vi "DualMotorControlExample.vi"() -> ()   [LabVIEW 2019, in "CubeMarsBLDClib.lvlib"]
uses:
  CubeMarsBLDClib.lvlib
  MotorParameters.ctl
  Reference.ctl
  MotorType.ctl
  ReadMotorData.ctl
  <vilib>/myRIO/Common/Instrument Driver Framework/myRIO v1.0/UART/vis/myRIO v1.0 Close UART.vi
  <vilib>/myRIO/Common/Instrument Driver Framework/Utilities/vis/FPGA Ref Manager.vi
  <vilib>/myRIO/Common/Instrument Driver Framework/myRIO v1.0/myRIO v1.0 Reset FPGA.vi
  <vilib>/myRIO/Common/Instrument Driver Framework/myRIO v1.0/IRQ/vis/myRIO v1.0 IRQ Info FGV.vi
  <vilib>/myRIO/Common/Instrument Driver Framework/myRIO v1.0/IRQ/vis/myRIO v1.0 Timer IRQ Info FGV.vi
  <vilib>/myRIO/Common/Instrument Driver Framework/myRIO v1.0/IRQ/vis/myRIO v1.0 ISR Agent.vi
  <vilib>/myRIO/Instrument Drivers/Utilities/vis/Reset Index.vi
  <vilib>/myRIO/Common/Instrument Driver Framework/myRIO v1.0/Resource Manager/vis/myRIO v1.0 Block Write Resource Manager.vi
  <vilib>/myRIO/Instrument Drivers/Utilities/Utilities.lvlib
panel:
  out "ReadData":T4(array[cluster])
  in  "Motor 1 CAN ID":u32=1
  in  "Enable Motor1":bool
  in  "Disable Motor1":bool
  in  "Motor1 ValueIn":T5
  out "FilteredValue":T5
  in  "Motor1 Send CMD":bool=TRUE
  in  "Motor 2 CAN ID":u32=2
  in  "Motor2 Send CMD":bool=TRUE
  out "FilteredValue":T5
  out "dt(ms)":dbl
  in  "Disable Motor2":bool
  in  "Motor2 ValueIn":T5
  in  "Enable Motor2":bool
  out "error out":errorcluster
  in  "stop":bool
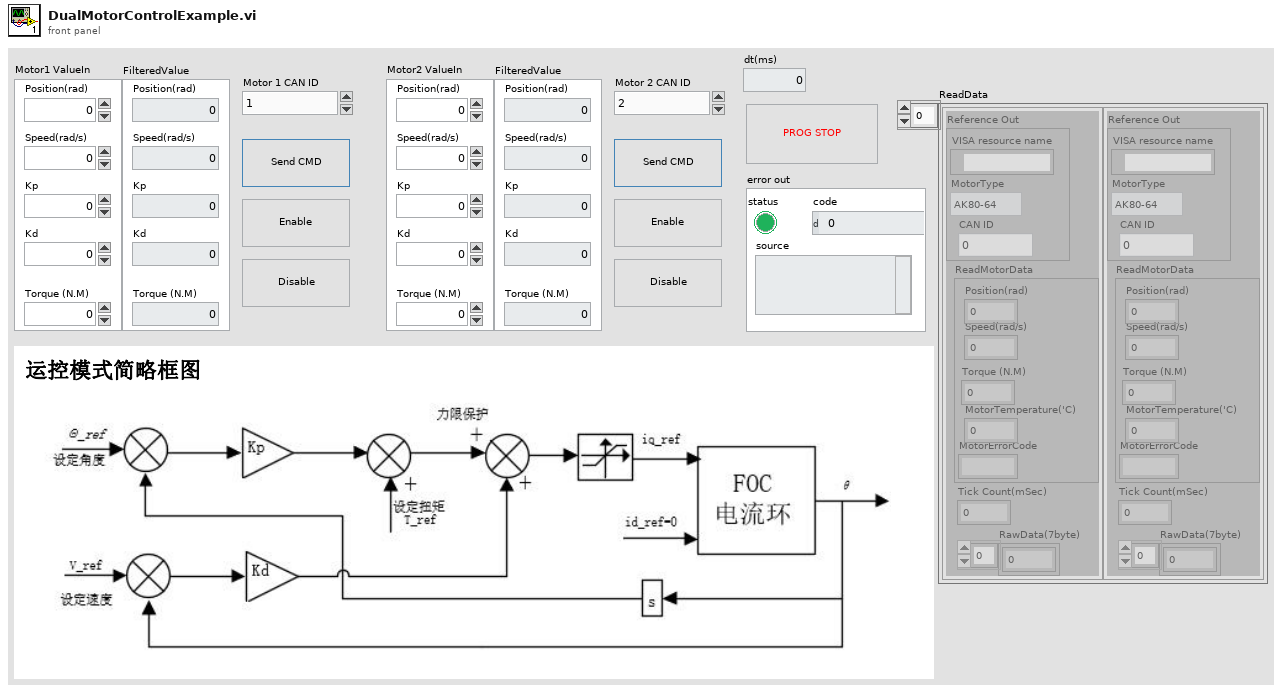
[diagram p1: front panel]
types:
  T1 = typedef "CubeMarsBLDClib.lvlib/Reference.ctl" = cluster{"VISA resource name":refnum<visa-resource-name>, "MotorType":T2, "CAN ID":u32}
  T2 = typedef "CubeMarsBLDClib.lvlib/MotorType.ctl" = enum16{"AK80-64", "AK80-9", "AK80-8", "AK80-6", "AK70-10", "AK60-6", "AK10-9"}
  T3 = typedef "CubeMarsBLDClib.lvlib/ReadMotorData.ctl" = cluster{"Position(rad)":dbl, "Speed(rad/s)":dbl, "Torque (N.M)":dbl, "MotorTemperature('C)":sgl, "MotorErrorCode":string}
  T4 = cluster{"Reference Out":T1, "ReadMotorData":T3, "Tick Count(mSec)":u32, "RawData(7byte)":u8[]}[]
  T5 = typedef "CubeMarsBLDClib.lvlib/MotorParameters.ctl" = cluster{"Position(rad)":dbl, "Speed(rad/s)":dbl, "Kp":dbl, "Kd":dbl, "Torque (N.M)":dbl}
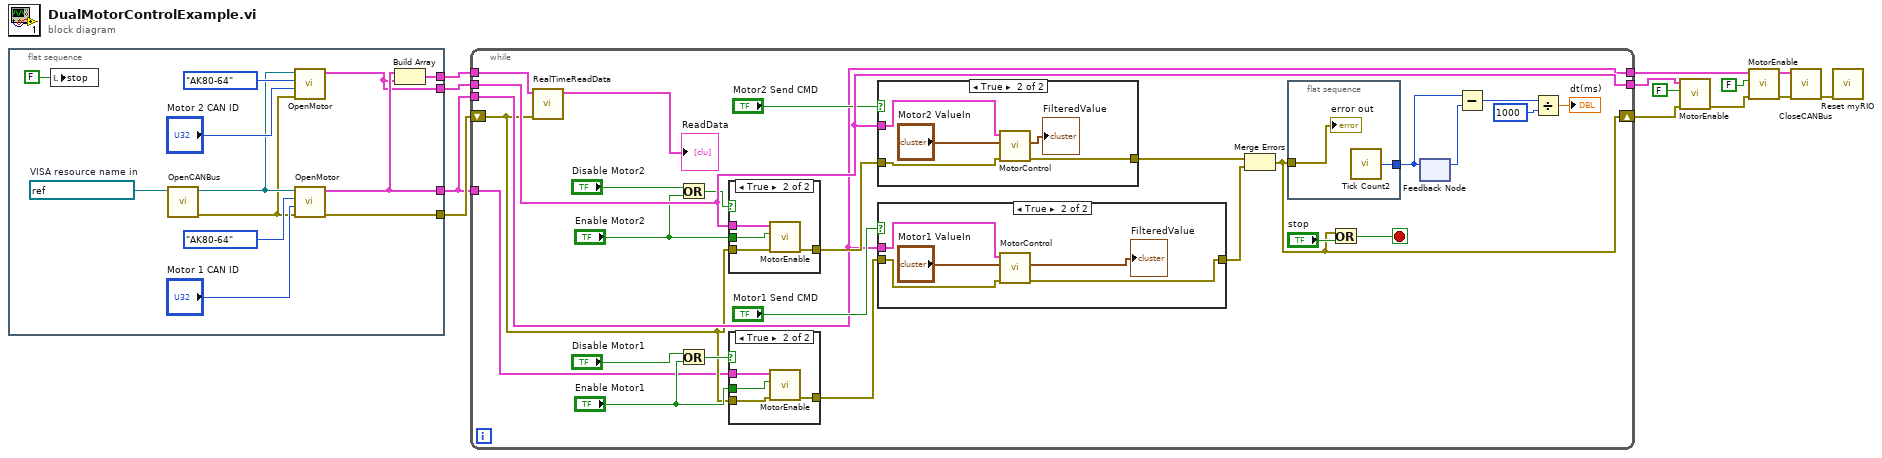
[diagram p0: block diagram]
diagram:
  n1 = flat-sequence {
    tunnel: [w15] -> w12
    tunnel: [w25] -> w3
    tunnel: [w21] -> w4
    tunnel: [w16] -> w2
    frame #0 {
      w22 = refnum<visa-resource-name> "ASRL3::INSTR"  # VISA resource name in
      n2 = local write "stop"(FALSE ("stop")) -> ()
      n3 = call "OpenCANBus.vi"("USB-CAN COM Port"=w22) -> ("Error Out"=w14:errorcluster, "VISA resource name out"=w17:refnum<visa-resource-name>)  [unwired: 9 in]
      n4 = call "OpenMotor.vi"("Error In"=w14, "CAN ID"="Motor 2 CAN ID", "MotorType"=MotorType."AK80-64", "USB CAN VISA resource name"=w17) -> ("Reference Out"=w15:T1)  [unwired: 6 in, 1 out]
      n5 = call "OpenMotor.vi"("Error In"=w14, "CAN ID"="Motor 1 CAN ID", "MotorType"=MotorType."AK80-64", "USB CAN VISA resource name"=w17) -> ("Error Out"=w21:errorcluster, "Reference Out"=w16:T1)  [unwired: 6 in]
      n6 = Build Array(w16, w15) -> (w25:T1[])
    }
  }
  n7 = while {
    shift-right: [w31] -> w11
    shift-left: w4 -> [w29]
    tunnel: w12 -> [w49]
    tunnel: [w49] -> w10
    tunnel: w2 -> [w34]
    tunnel: w2 -> [w27]
    tunnel: [w34] -> w7
    tunnel: w3 -> [w28]
    stop <- w50 stop-if-true
    n8 = call "RealTimeReadData.vi"("error in"=w29, "AllMotorReference(Same port)"=w28) -> ("ReadData"=→"ReadData":T4)  [unwired: 8 in, 1 out]
    n9 = Or(x="Disable Motor2", y="Enable Motor2") -> (x .or. y?=w46:bool)
    n10 = Or(x="Disable Motor1", y="Enable Motor1") -> (x .or. y?=w41:bool)
    n11 = case shown="True" w46 {
      tunnel: w29 -> [w71 w75]
      tunnel: [w71 w74] -> w44
      tunnel: w49 -> [_ w73]
      tunnel: "Enable Motor2" -> [_ w72]
      frame False {
      }
      frame True {
        n12 = call "MotorEnable.vi"("Error In"=w75, "Enable?(F)"=w72, "Reference In"=w73) -> ("Error Out"=w74:errorcluster)  [unwired: 7 in, 1 out]
      }
    }
    n13 = case shown="True" w41 {
      tunnel: w29 -> [w60 w64]
      tunnel: [w60 w63] -> w43
      tunnel: w27 -> [_ w62]
      tunnel: "Enable Motor1" -> [_ w61]
      frame False {
      }
      frame True {
        n14 = call "MotorEnable.vi"("Error In"=w64, "Enable?(F)"=w61, "Reference In"=w62) -> ("Error Out"=w63:errorcluster)  [unwired: 7 in, 1 out]
      }
    }
    n15 = case shown="True" "Motor2 Send CMD" {
      tunnel: [w65 w70] -> w33
      tunnel: w44 -> [w65 w69]
      tunnel: w49 -> [_ w68]
      frame False {
      }
      frame True {
        n16 = call "MotorControl.vi"("error in"=w69, "ValueIn"="Motor2 ValueIn", "Reference In"=w68) -> ("error out"=w70:errorcluster, "FilteredValue"=→"FilteredValue":T5)  [unwired: 6 in, 1 out]
      }
    }
    n17 = case shown="True" "Motor1 Send CMD" {
      tunnel: [w54 w59] -> w32
      tunnel: w43 -> [w54 w58]
      tunnel: w34 -> [_ w57]
      frame False {
      }
      frame True {
        n18 = call "MotorControl.vi"("error in"=w58, "ValueIn"="Motor1 ValueIn", "Reference In"=w57) -> ("error out"=w59:errorcluster, "FilteredValue"=→"FilteredValue":T5)  [unwired: 6 in, 1 out]
      }
    }
    n19 = Merge Errors(w33, w32) -> (w31:errorcluster)
    n20 = flat-sequence {
      tunnel: [w53] -> w37
      tunnel: w31 -> [w52]
      frame #0 {
        n21 = call "Tick Count2"() -> ("Tick Count(uSec)"=w53:u32)
        "error out" <- w52
      }
    }
    n22 = Or(x=w31, y="stop") -> (x .or. y?=w50:bool)
    n23 = feedback #1() -> (w38:u32)  [unwired: 1 in]
    n24 = feedback-in #1(w37) -> ()
    n25 = Subtract(x=w37, y=w38) -> (x-y=w39:u32)
    n26 = Divide(x=w39, y=u32 1000) -> (x/y=→"dt(ms)":dbl)
  }
  n27 = call "MotorEnable.vi"("Error In"=w11, "Enable?(F)"=FALSE, "Reference In"=w10) -> ("Error Out"=w6:errorcluster)  [unwired: 7 in, 1 out]
  n28 = call "MotorEnable.vi"("Error In"=w6, "Enable?(F)"=FALSE, "Reference In"=w7) -> ("Error Out"=w1:errorcluster, "Reference Out"=w5:T1)  [unwired: 7 in]
  n29 = call "CloseCANBus.vi"("Error In"=w1, "Reference In"=w5) -> ("Error Out"=w13:errorcluster)  [unwired: 9 in]
  n30 = call <vilib>:"Reset myRIO.vi"("error in (no error)"=w13) -> ()  [unwired: 10 in, 1 out]
